vi "TDS Comms Disconnect.vi"(8 "error in (no error)":errorcluster, 11 "Address":string) -> (0 "error out":errorcluster)   [LabVIEW 2025, in "Interface Functions.lvlib"]
uses:
  Interface Functions.lvlib
panel:
  # "Comms Disconnect"
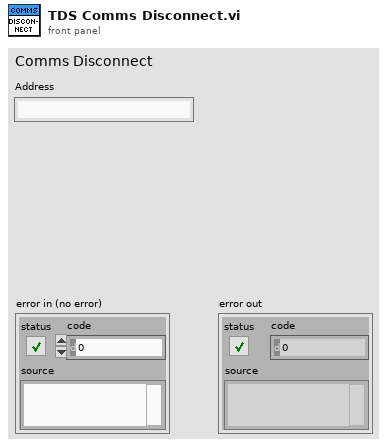
[diagram p1: front panel]
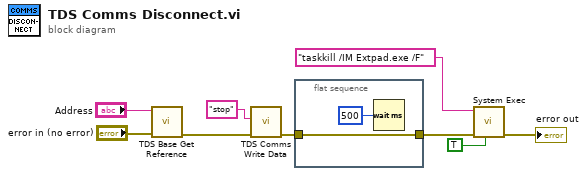
[diagram p0: block diagram]
diagram:
  n1 = call "TDS Base Get Reference.vi"("error in (no error)"="error in (no error)", "Address"="Address") -> ("error out"=w2:errorcluster)  [unwired: 8 in, 1 out]
  n2 = call "TDS Comms Write Data.vi"("error in (no error)"=w2, "Write Data"="stop") -> ("error out"=w4:errorcluster)  [unwired: 8 in, 1 out]
  n3 = flat-sequence {
    tunnel: [w10] -> w3
    tunnel: w4 -> [w10]
    frame #0 {
      n4 = Wait (ms)(milliseconds to wait=u32 500) -> ()  [unwired: 1 out]
    }
  }
  n5 = call <vilib>:"System Exec.vi"("run minimized? (F)"=TRUE, "error in (no error)"=w3, "command line"="taskkill /IM Extpad.exe /F") -> ("error out"=→"error out":errorcluster)  [unwired: 5 in, 3 out]
